vi "Configure Counter Frequency.vi"(7 "Trigger Level (0)":dbl, 8 "error in (no error)":errorcluster, 9 "Enable Counter Frequency (F: Disable)":bool, 10 "Channel Name (0: Channel 1)":i32(ring) items=["Channel 1", "Channel 2"], 11 "VISA resource name":refnum<visa-resource-name>) -> (0 "error out":errorcluster, 3 "VISA resource name out":refnum<visa-resource-name>)   [LabVIEW 2017, in "Tektronix TDS 200 1000 2000 Series.lvlib"]
doc: "Configures the counter frequency.\n\n<B>Note(s):</b>\nAvailable on TBS1000B-EDU and TBS1000B series only."
uses:
  Tektronix TDS 200 1000 2000 Series.lvlib
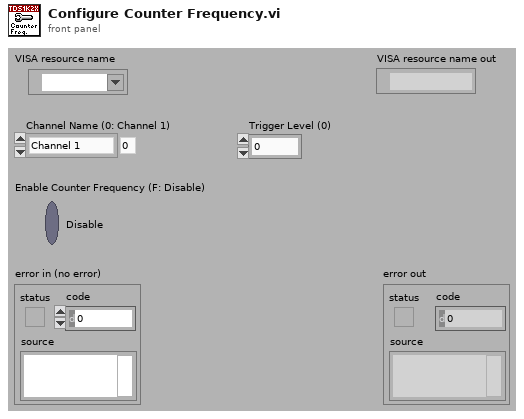
[diagram p1: front panel]
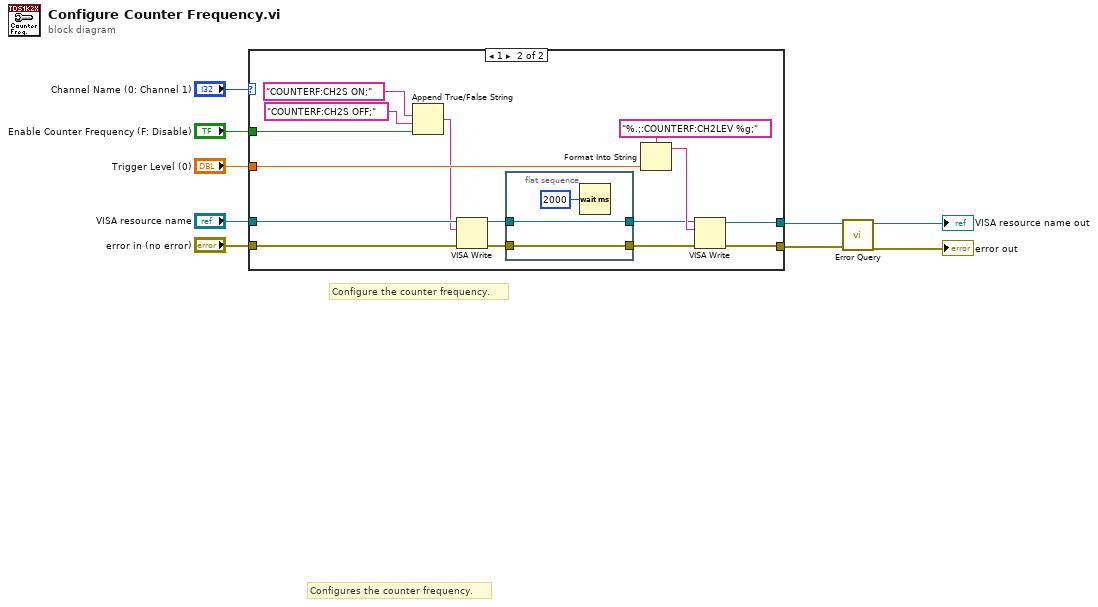
[diagram p0: block diagram]
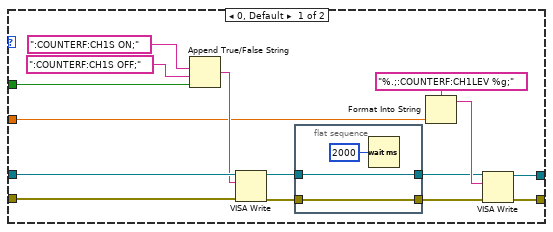
[diagram p2: hidden frame]
diagram:
  # "Configure the counter frequency."
  # "Configures the counter frequency."
  n1 = case shown="1" "Channel Name (0: Channel 1)" {
    tunnel: "Enable Counter Frequency (F: Disable)" -> [w21 w40]
    tunnel: "Trigger Level (0)" -> [w14 w38]
    tunnel: "VISA resource name" -> [w17 w35]
    tunnel: "error in (no error)" -> [w16 w34]
    tunnel: [w19 w36] -> w2
    tunnel: [w18 w28] -> w1
    frame 0, Default {
      n2 = Append True/False String(1:w21, 2:":COUNTERF:CH1S OFF;", 3:":COUNTERF:CH1S ON;") -> (0:w15:string)  [unwired: 1 out]
      n3 = VISA Write(VISA resource name=w17, write buffer=w15, error in (no error)=w16) -> (VISA resource name out=w13:refnum<visa-resource-name>, error out=w10:errorcluster)  [unwired: 1 out]
      n4 = flat-sequence {
        tunnel: w13 -> [w27]
        tunnel: [w27] -> w12
        tunnel: [w26] -> w11
        tunnel: w10 -> [w26]
        frame #0 {
          n5 = Wait (ms)(milliseconds to wait=u32 2000) -> ()  [unwired: 1 out]
        }
      }
      n6 = Format Into String(format string="%.;:COUNTERF:CH1LEV %g;", w14) -> (resulting string=w20:string)  [unwired: 2 in, 1 out]
      n7 = VISA Write(VISA resource name=w12, write buffer=w20, error in (no error)=w11) -> (VISA resource name out=w19:refnum<visa-resource-name>, error out=w18:errorcluster)  [unwired: 1 out]
    }
    frame 1 {
      n8 = Append True/False String(1:w40, 2:"COUNTERF:CH2S OFF;", 3:"COUNTERF:CH2S ON;") -> (0:w33:string)  [unwired: 1 out]
      n9 = VISA Write(VISA resource name=w35, write buffer=w33, error in (no error)=w34) -> (VISA resource name out=w32:refnum<visa-resource-name>, error out=w31:errorcluster)  [unwired: 1 out]
      n10 = flat-sequence {
        tunnel: w32 -> [w45]
        tunnel: [w45] -> w30
        tunnel: [w44] -> w29
        tunnel: w31 -> [w44]
        frame #0 {
          n11 = Wait (ms)(milliseconds to wait=u32 2000) -> ()  [unwired: 1 out]
        }
      }
      n12 = Format Into String(format string="%.;:COUNTERF:CH2LEV %g;", w38) -> (resulting string=w37:string)  [unwired: 2 in, 1 out]
      n13 = VISA Write(VISA resource name=w30, write buffer=w37, error in (no error)=w29) -> (VISA resource name out=w36:refnum<visa-resource-name>, error out=w28:errorcluster)  [unwired: 1 out]
    }
  }
  n14 = call "Error Query.vi"("error in (no error)"=w1, "VISA resource name"=w2) -> ("error out"=→"error out":errorcluster, "VISA resource name out"=→"VISA resource name out":refnum<visa-resource-name>)  [unwired: 8 out]
